vi "cRIO Main.vi"() -> ()   [LabVIEW 2021]
uses:
  <vilib>/NI/LVFPGA Adv Session Resources/ResourceInfo.ctl
  <vilib>/FPGAPlugInAG/cRIO-9053/niLvFpga_Open_cRIO-9053.vi
  <vilib>/rvi/interface/common/dynamic/niFpgaDynamicAddResources.vi
  <vilib>/Utility/error.llb/Error Cluster From Error Code.vi
  <vilib>/rvi/errors/niLvFpgaAdjustHostInterfaceError.vi
  <vilib>/FPGAPlugInAG/Dynamic/niLvFpga_Close_Dynamic.vi
  <vilib>/rvi/interface/nirviOpenFPGA/nirviOpenFPGA.xnode
  FPGA Bitfiles/fpga-bus_FPGATarget_ExampleFPGAMain.lvbitx
  <vilib>/rvi/interface/nirviReadWriteControl/nirviReadWriteControl.xnode
  <vilib>/rvi/interface/nirviCloseFPGA/nirviCloseFPGA.xnode
  <vilib>/NI/LVFPGA Adv Session Resources/LVFPGAAdvSessionResources.lvlib
  <vilib>/rvi/interface/Simulation/niFpgaSimulationCallBeginRW.vi
  NiFpgaLv.dll
panel:
  in  "stop 2":bool
  out "I64 Out":i64
  in  "I64":i64
  out "Resource info out":T1[](array[typedef])
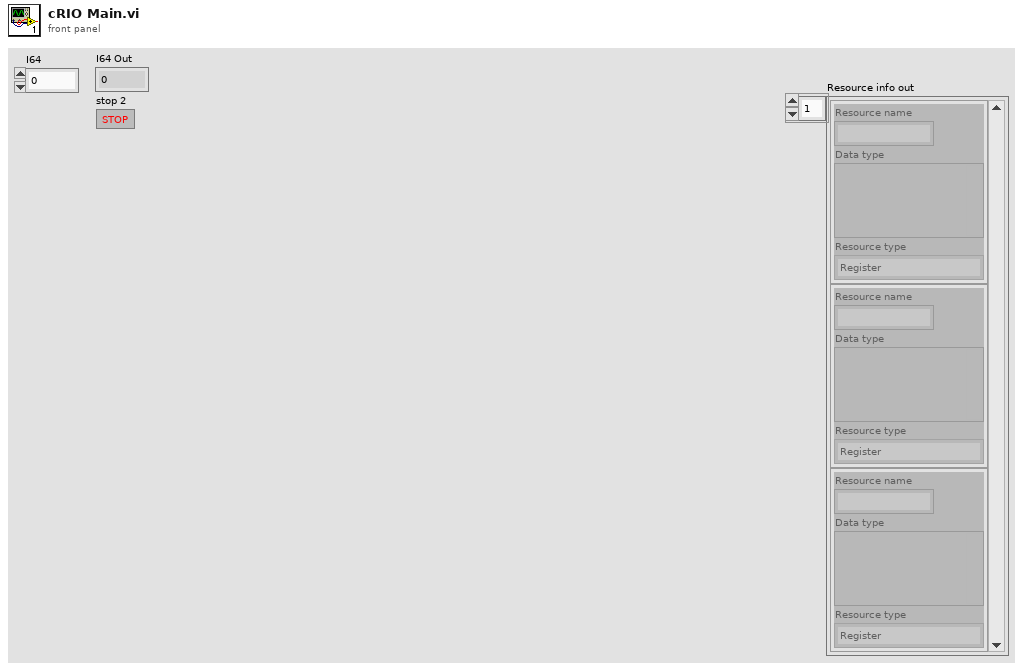
[diagram p1: front panel]
types:
  T1 = typedef "LVFPGAAdvSessionResources.lvlib/ResourceInfo.ctl" = cluster{"Resource name":string, "Data type":variant, "Resource type":enum16{"Register", "Host To Target FIFO", "Target To Host FIFO"}}
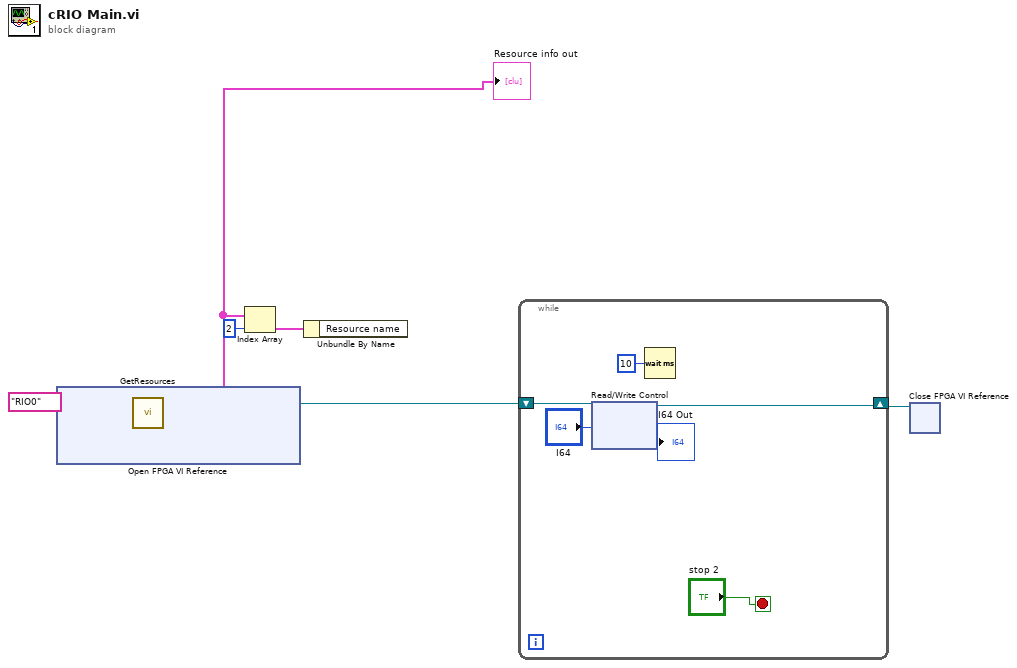
[diagram p0: block diagram]
diagram:
  n1 = xnode "Open FPGA VI Reference"("resource name"=tag "RIO0") -> ("FPGA VI Reference Out"=w6:refnum<k20>)  [unwired: 1 in, 1 out]
  n2 = call <vilib>:"GetResources.vi"("FPGA VI Reference in"=w6) -> ("Resource info out"=w4:T1[], "FPGA VI Reference out"=w5:refnum<k20>)  [unwired: 8 in, 1 out]
  "Resource info out" <- w4
  n3 = Index Array(array=w4, index=2) -> (element=w2:T1)
  n4 = Unbundle By Name(w2) -> ()  [unwired: 1 out]
  n5 = while {
    shift-right: [w12] -> w1
    shift-left: w5 -> [w13]
    stop <- "stop 2" stop-if-true
    n6 = xnode "Read/Write Control"("FPGA VI Reference In"=w13, "I64 Value"="I64") -> ("FPGA VI Reference Out"=w12:refnum<k20>, "I64 Out"=→"I64 Out":i64)  [unwired: 1 in, 1 out]
    n7 = Wait (ms)(milliseconds to wait=u32 10) -> ()  [unwired: 1 out]
  }
  n8 = xnode "Close FPGA VI Reference"("FPGA VI Reference In"=w1) -> ()  [unwired: 1 in, 1 out]
